vi "GetContourResultName.vi"(7 "ProjectName":string, 11 "ROIName":string) -> (3 "ContourResultName":string[](array[string]))   [LabVIEW 2019]
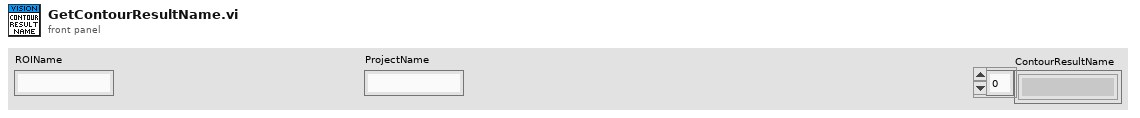
[diagram p1: front panel]
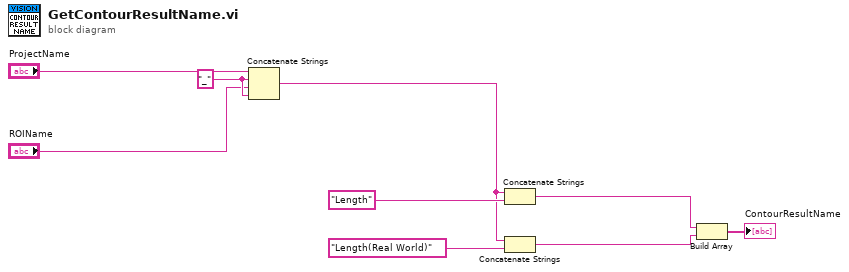
[diagram p0: block diagram]
diagram:
  w9 = "_" ("string")
  n1 = Concatenate Strings("ProjectName", w9, "ROIName", w9) -> (w4:string)
  n2 = Concatenate Strings(w4, "Length") -> (w3:string)
  n3 = Concatenate Strings(w4, "Length(Real World)") -> (w2:string)
  n4 = Build Array(w3, w2) -> (→"ContourResultName":string[])
